vi "PeriodicFilter-Format L1 Info String.vi"(10 "Time format string":string="%<%H:%M:%S%3u>T", 11 "entry":T1[](array[typedef])) -> (3 "Array":string[](array[string]))   [LabVIEW 2017, in "Communicable State Machine.lvlib"]
uses:
  Communicable State Machine.lvlib
  Periodic String Filter Info.ctl
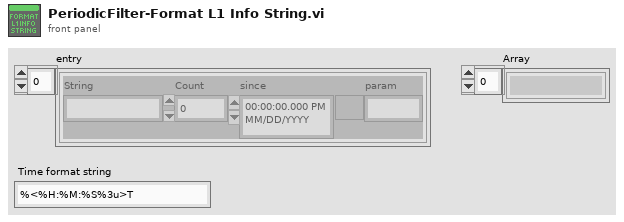
[diagram p1: front panel]
types:
  T1 = typedef "Communicable State Machine.lvlib/Periodic String Filter Info.ctl" = cluster{"String":string, "Count":i64, "since":timestamp, "param":string}
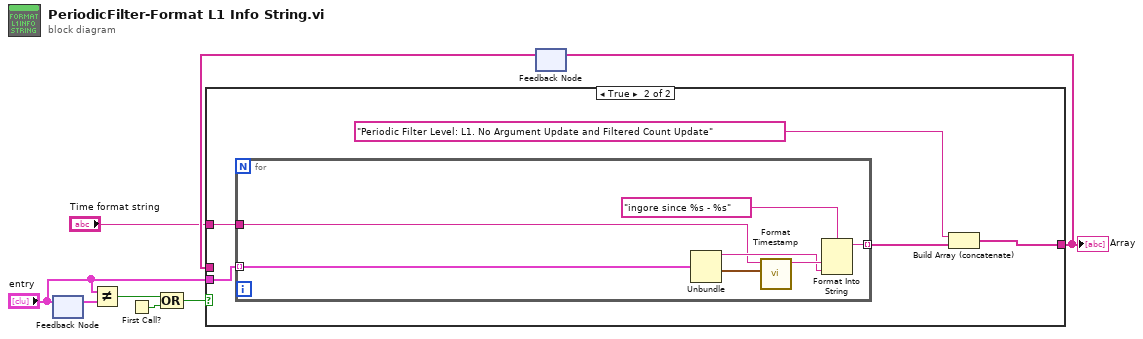
[diagram p0: block diagram]
diagram:
  n1 = feedback #1() -> (w5:T1[])  [unwired: 1 in]
  n2 = feedback-in #1("entry") -> ()
  n3 = Not Equal?(x="entry", y=w5) -> (x != y?=w6:bool)
  n4 = First Call?() -> (First Call?: T/F=w7:bool)
  n5 = Compound Arithmetic op=OR(w6, w7) -> (w4:bool)
  n6 = feedback #2() -> (w8:string[])  [unwired: 1 in]
  n7 = case shown="True" w4 {
    tunnel: [w9 w11] -> w2
    tunnel: "entry" -> [_ w13]
    tunnel: w8 -> [w9 _]
    tunnel: "Time format string" -> [_ w12]
    frame False {
    }
    frame True {
      n8 = for {
        tunnel: w13 -> [w20] mode=indexing
        tunnel: [w21] -> w14 mode=indexing
        tunnel: w12 -> [w15]
        n9 = Unbundle(w20) -> ("String"=w16:string, "since"=w18:timestamp)  [unwired: 2 out]
        n10 = call "Format Timestamp.vi"("timestamp"=w18, "format string"=w15) -> ("String"=w17:string)  [unwired: 9 in]
        n11 = Format Into String(format string="ingore since %s - %s", w17, w16) -> (resulting string=w21:string)  [unwired: 2 in, 1 out]
      }
      n12 = Build Array (concatenate)("Periodic Filter Level: L1. No Argument Update and Filtered Count Update" ("format string"), w14) -> (w11:string[])
    }
  }
  "Array" <- w2
  n13 = feedback-in #2(w2) -> ()
